vi "PathPlanner_Path_Equals.vi"(9 "Other Path":T1={"BezierPoints"=[], "PreviewStartingRotation"={"VALUE"=0.0, "COS"=1.0, "SIN"=0.0}, "Reversed"=FALSE, "RotationTargets"=[], "ConstraintZones"=[], "EventMarkers"=[], "GlobalConstraints"={"MaxVelocityMps;"=0.0, "MaxAccelerationMpsSq;"=0.0, "MaxAngularVelRadPsEc;"=0.0, "MaxAngularAccRadPSecSq"=0.0, "Exists"=FALSE}, "GoalEndState"={"Velocity"=0.0, "Rotation"={"VALUE"=0.0, "COS"=1.0, "SIN"=0.0}}, "AllPoints"=[]} {"AllPoints"."HolonomicRotation"."SIN" format="%13.4f"; "AllPoints"."HolonomicRotation"."COS" format="%13.4f"; "AllPoints"."HolonomicRotation"."VALUE" format="%13.4f"; "AllPoints"."Position"."Y" format="%14.3f"; "AllPoints"."Position"."X" format="%14.3f"; "GoalEndState"."Rotation"."SIN" format="%13.4f"; "GoalEndState"."Rotation"."COS" format="%13.4f"; "GoalEndState"."Rotation"."VALUE" format="%13.4f"; "EventMarkers"."lastRobotPos"."Y" format="%14.3f"; "EventMarkers"."lastRobotPos"."X" format="%14.3f"; "EventMarkers"."markerPos"."Y" format="%14.3f"; "EventMarkers"."markerPos"."X" format="%14.3f"; "RotationTargets"."target"."SIN" format="%13.4f"; "RotationTargets"."target"."COS" format="%13.4f"; "RotationTargets"."target"."VALUE" format="%13.4f"; "PreviewStartingRotation"."SIN" format="%13.4f"; "PreviewStartingRotation"."COS" format="%13.4f"; "PreviewStartingRotation"."VALUE" format="%13.4f"; "BezierPoints"."Y" format="%14.3f"; "BezierPoints"."X" format="%14.3f"}, 11 "Path":T1={"BezierPoints"=[], "PreviewStartingRotation"={"VALUE"=0.0, "COS"=1.0, "SIN"=0.0}, "Reversed"=FALSE, "RotationTargets"=[], "ConstraintZones"=[], "EventMarkers"=[], "GlobalConstraints"={"MaxVelocityMps;"=0.0, "MaxAccelerationMpsSq;"=0.0, "MaxAngularVelRadPsEc;"=0.0, "MaxAngularAccRadPSecSq"=0.0, "Exists"=FALSE}, "GoalEndState"={"Velocity"=0.0, "Rotation"={"VALUE"=0.0, "COS"=1.0, "SIN"=0.0}}, "AllPoints"=[]} {"AllPoints"."HolonomicRotation"."SIN" format="%13.4f"; "AllPoints"."HolonomicRotation"."COS" format="%13.4f"; "AllPoints"."HolonomicRotation"."VALUE" format="%13.4f"; "AllPoints"."Position"."Y" format="%14.3f"; "AllPoints"."Position"."X" format="%14.3f"; "GoalEndState"."Rotation"."SIN" format="%13.4f"; "GoalEndState"."Rotation"."COS" format="%13.4f"; "GoalEndState"."Rotation"."VALUE" format="%13.4f"; "EventMarkers"."lastRobotPos"."Y" format="%14.3f"; "EventMarkers"."lastRobotPos"."X" format="%14.3f"; "EventMarkers"."markerPos"."Y" format="%14.3f"; "EventMarkers"."markerPos"."X" format="%14.3f"; "RotationTargets"."target"."SIN" format="%13.4f"; "RotationTargets"."target"."COS" format="%13.4f"; "RotationTargets"."target"."VALUE" format="%13.4f"; "PreviewStartingRotation"."SIN" format="%13.4f"; "PreviewStartingRotation"."COS" format="%13.4f"; "PreviewStartingRotation"."VALUE" format="%13.4f"; "BezierPoints"."Y" format="%14.3f"; "BezierPoints"."X" format="%14.3f"}) -> (3 "Equals":bool)   [LabVIEW 2019, in "PathPlanner24.lvlib"]
doc: "NOT DONE - DONT USE"
uses:
  PathPlanner24.lvlib
  <vilib>/Rock Robotics/WPI/ThirdParty/JAS_Junk/TrajLib/Trajectory_Library.lvlib
  <vilib>/Rock Robotics/WPI/ThirdParty/JAS_Junk/TrajLib/TypeDef/TRANSLATION2D.ctl
  <vilib>/Rock Robotics/WPI/ThirdParty/JAS_Junk/TrajLib/TypeDef/ROTATION2D.ctl
  TypeDef/PathPlannerRotationTarget.ctl
  TypeDef/PathPlannerPathConstraints.ctl
  TypeDef/PathPlannerConstraintsZone.ctl
  TypeDef/PathPlannerCommandUtil.ctl
  TypeDef/PathPlannerEventMarker.ctl
  TypeDef/PathPlannerGoalEndState.ctl
  TypeDef/PathPlannerPathPoint.ctl
  TypeDef/PathPlannerPath.ctl
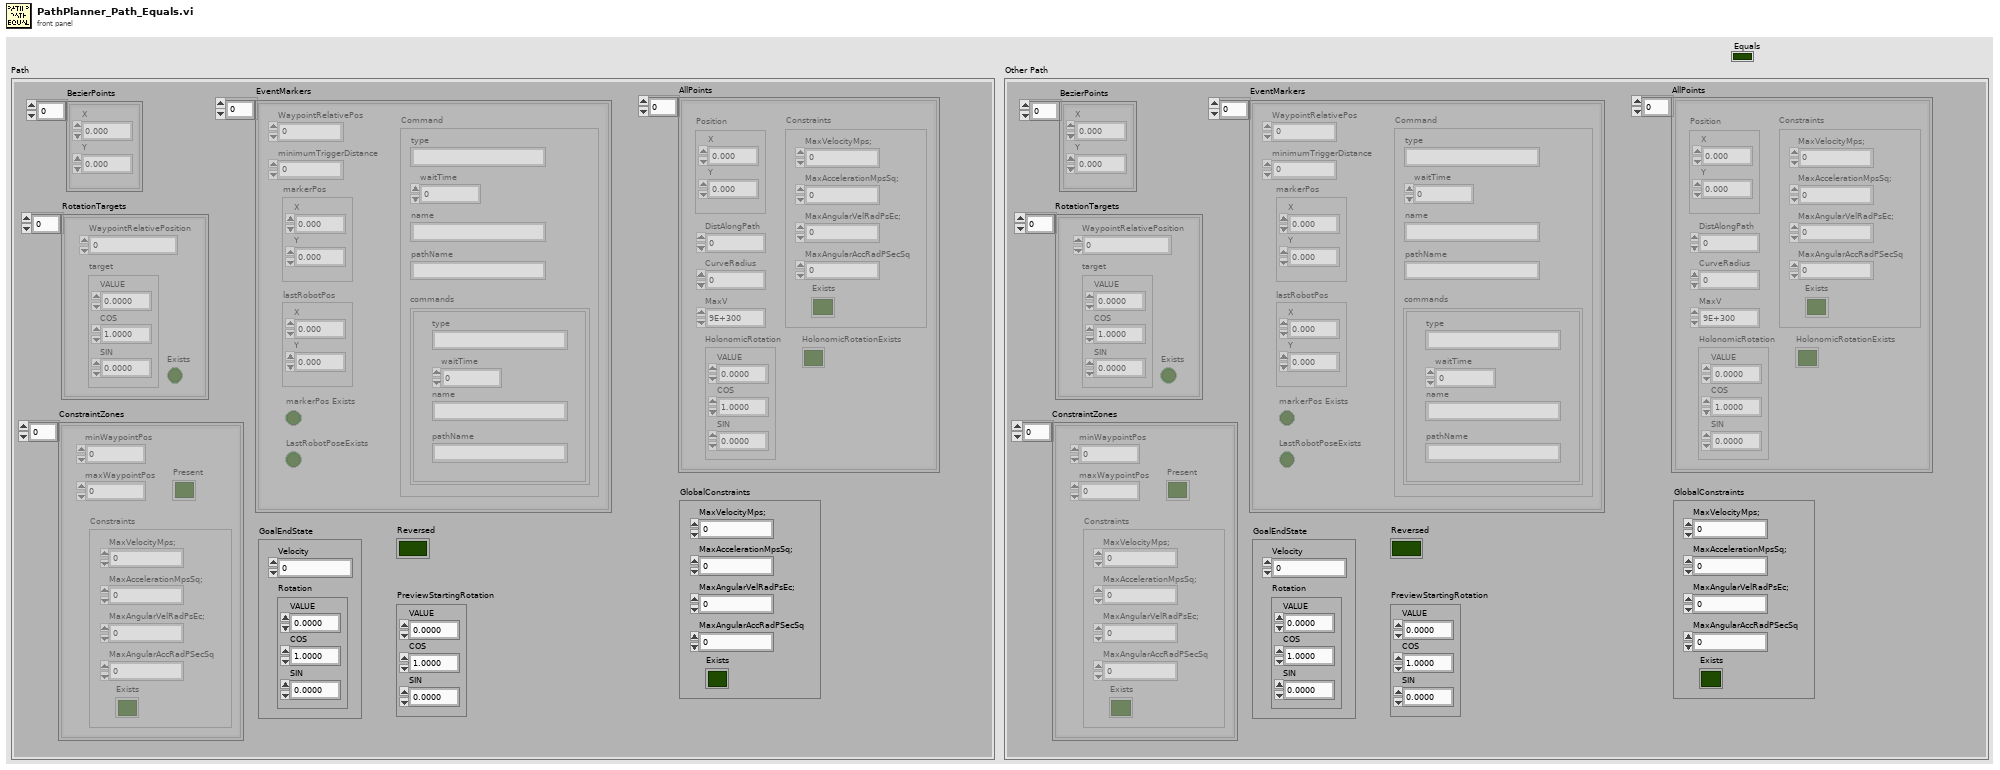
[diagram p1: front panel]
types:
  T1 = typedef "PathPlanner24.lvlib/PathPlannerPath.ctl" = cluster{"BezierPoints":T2[], "PreviewStartingRotation":T3, "Reversed":bool, "RotationTargets":T4[], "ConstraintZones":T5[], "EventMarkers":T7[], "GlobalConstraints":T6, "GoalEndState":T9, "AllPoints":T10[]}
  T2 = typedef "Trajectory_Library.lvlib/TRANSLATION2D.ctl" = cluster{"X":dbl, "Y":dbl}
  T3 = typedef "Trajectory_Library.lvlib/ROTATION2D.ctl" = cluster{"VALUE":dbl, "COS":dbl, "SIN":dbl}
  T4 = typedef "PathPlanner24.lvlib/PathPlannerRotationTarget.ctl" = cluster{"target":T3, "WaypointRelativePosition":dbl, "Exists":bool}
  T5 = typedef "PathPlanner24.lvlib/PathPlannerConstraintsZone.ctl" = cluster{"minWaypointPos":dbl, "maxWaypointPos":dbl, "Constraints":T6, "Present":bool}
  T6 = typedef "PathPlanner24.lvlib/PathPlannerPathConstraints.ctl" = cluster{"MaxVelocityMps;":dbl, "MaxAccelerationMpsSq;":dbl, "MaxAngularVelRadPsEc;":dbl, "MaxAngularAccRadPSecSq":dbl, "Exists":bool}
  T7 = typedef "PathPlanner24.lvlib/PathPlannerEventMarker.ctl" = cluster{"WaypointRelativePos":dbl, "minimumTriggerDistance":dbl, "markerPos":T2, "lastRobotPos":T2, "Command":T8, "markerPos Exists":bool, "LastRobotPoseExists":bool}
  T8 = typedef "PathPlanner24.lvlib/PathPlannerCommandUtil.ctl" = cluster{"waitTime":dbl, "name":string, "type":string, "pathName":string, "commands":cluster{"type":string, "waitTime":dbl, "name":string, "pathName":string}[]}
  T9 = typedef "PathPlanner24.lvlib/PathPlannerGoalEndState.ctl" = cluster{"Velocity":dbl, "Rotation":T3}
  T10 = typedef "PathPlanner24.lvlib/PathPlannerPathPoint.ctl" = cluster{"Position":T2, "HolonomicRotation":T3, "DistAlongPath":dbl, "CurveRadius":dbl, "MaxV":dbl, "Constraints":T6, "HolonomicRotationExists":bool}
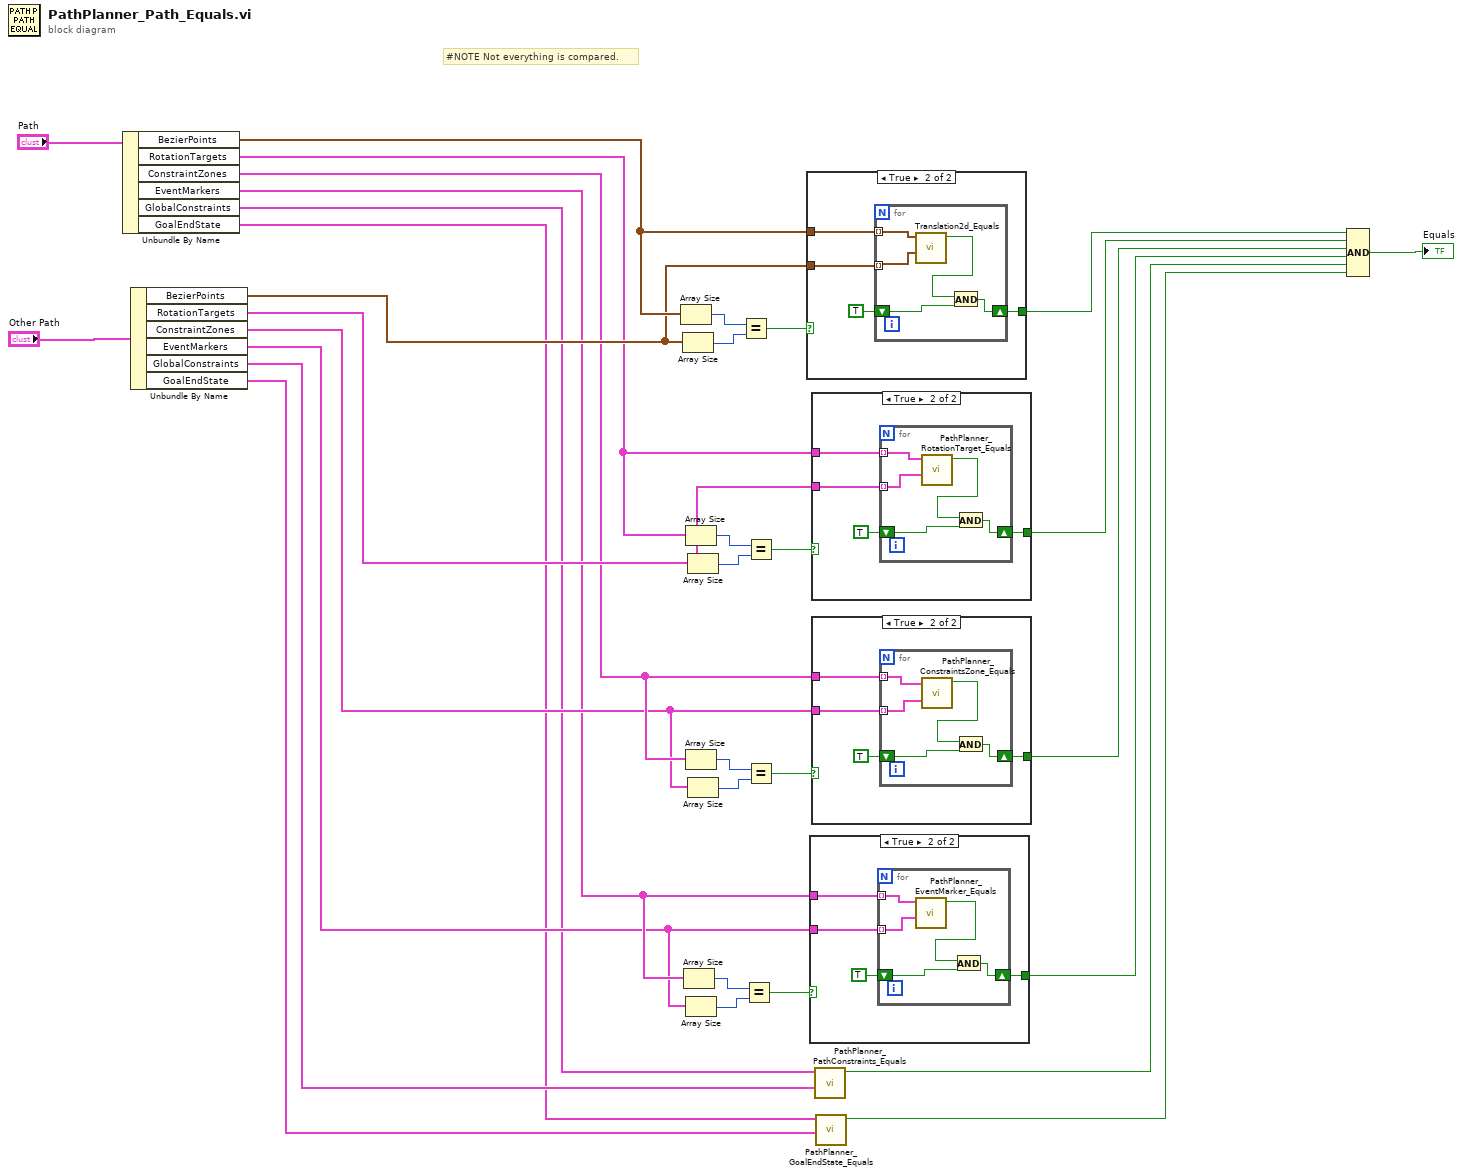
[diagram p0: block diagram]
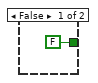
[diagram p2: hidden frame]
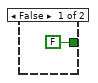
[diagram p3: hidden frame]
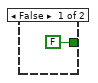
[diagram p4: hidden frame]
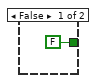
[diagram p5: hidden frame]
diagram:
  # "#NOTE Not everything is compared."
  n1 = Unbundle By Name("Path") -> ("BezierPoints"=w28:T2[], "RotationTargets"=w21:T4[], "ConstraintZones"=w15:T5[], "EventMarkers"=w9:T7[], "GlobalConstraints"=w6:T6, "GoalEndState"=w3:T9)
  n2 = Unbundle By Name("Other Path") -> ("BezierPoints"=w27:T2[], "RotationTargets"=w20:T4[], "ConstraintZones"=w14:T5[], "EventMarkers"=w8:T7[], "GlobalConstraints"=w5:T6, "GoalEndState"=w2:T9)
  n3 = Array Size(array=w28) -> (size(s)=w31:i32)
  n4 = Array Size(array=w27) -> (size(s)=w30:i32)
  n5 = Array Size(array=w9) -> (size(s)=w12:i32)
  n6 = Array Size(array=w21) -> (size(s)=w24:i32)
  n7 = Array Size(array=w15) -> (size(s)=w18:i32)
  n8 = Array Size(array=w8) -> (size(s)=w11:i32)
  n9 = Array Size(array=w20) -> (size(s)=w23:i32)
  n10 = Array Size(array=w14) -> (size(s)=w17:i32)
  n11 = Equal?(x=w31, y=w30) -> (x = y?=w29:bool)
  n12 = Equal?(x=w12, y=w11) -> (x = y?=w10:bool)
  n13 = Equal?(x=w24, y=w23) -> (x = y?=w22:bool)
  n14 = Equal?(x=w18, y=w17) -> (x = y?=w16:bool)
  n15 = case shown="True" w29 {
    tunnel: w28 -> [_ w37]
    tunnel: w27 -> [_ w36]
    tunnel: [FALSE w35] -> w26
    frame False {
    }
    frame True {
      n16 = for {
        shift-right: [w43] -> w35
        shift-left: TRUE -> [w42]
        tunnel: w37 -> [w41] mode=indexing
        tunnel: w36 -> [w40] mode=indexing
        n17 = call <vilib>:"Translation2d_Equals.vi"("other Translation"=w40, "In Translation"=w41) -> ("Equals"=w39:bool)  [unwired: 9 in]
        n18 = And(x=w39, y=w42) -> (x .and. y?=w43:bool)
      }
    }
  }
  n19 = case shown="True" w10 {
    tunnel: w9 -> [_ w47]
    tunnel: w8 -> [_ w46]
    tunnel: [FALSE w45] -> w7
    frame False {
    }
    frame True {
      n20 = for {
        shift-right: [w53] -> w45
        shift-left: TRUE -> [w52]
        tunnel: w47 -> [w51] mode=indexing
        tunnel: w46 -> [w50] mode=indexing
        n21 = call "PathPlanner_EventMarker_Equals.vi"("Other EventMarker"=w50, "EventMarker"=w51) -> ("Equal"=w49:bool)  [unwired: 9 in]
        n22 = And(x=w49, y=w52) -> (x .and. y?=w53:bool)
      }
    }
  }
  n23 = case shown="True" w22 {
    tunnel: w21 -> [_ w57]
    tunnel: w20 -> [_ w56]
    tunnel: [FALSE w55] -> w19
    frame False {
    }
    frame True {
      n24 = for {
        shift-right: [w63] -> w55
        shift-left: TRUE -> [w62]
        tunnel: w57 -> [w61] mode=indexing
        tunnel: w56 -> [w60] mode=indexing
        n25 = call "PathPlanner_RotationTarget_Equals.vi"("Other GoalEndState"=w60, "RotationTarget"=w61) -> ("Equal"=w59:bool)  [unwired: 9 in]
        n26 = And(x=w59, y=w62) -> (x .and. y?=w63:bool)
      }
    }
  }
  n27 = case shown="True" w16 {
    tunnel: w15 -> [_ w67]
    tunnel: w14 -> [_ w66]
    tunnel: [FALSE w65] -> w13
    frame False {
    }
    frame True {
      n28 = for {
        shift-right: [w73] -> w65
        shift-left: TRUE -> [w72]
        tunnel: w67 -> [w71] mode=indexing
        tunnel: w66 -> [w70] mode=indexing
        n29 = call "PathPlanner_ConstraintsZone_Equals.vi"("Other Constraints Zone"=w70, "ConstraintsZone"=w71) -> ("Equal"=w69:bool)  [unwired: 9 in]
        n30 = And(x=w69, y=w72) -> (x .and. y?=w73:bool)
      }
    }
  }
  n31 = call "PathPlanner_PathConstraints_Equals.vi"("Other PathPlannerConstraints"=w5, "PathPlannerConstraints"=w6) -> ("Equal"=w4:bool)  [unwired: 9 in]
  n32 = call "PathPlanner_GoalEndState_Equals.vi"("Other GoalEndState"=w2, "GoalEndState"=w3) -> ("Equal"=w1:bool)  [unwired: 9 in]
  n33 = Compound Arithmetic op=AND(w26, w19, w13, w7, w4, w1) -> (→"Equals":bool)
